vi "Code Complexity String.vi"(11 "CodeComplexity":sgl) -> (3 "Code Complexity String":string)   [LabVIEW 2023, in "VIDoc Printer.lvlib" / "VIDoc Printer.lvclass"]
doc: "Converts the Code Complexity value into a printable String."
uses:
  VIDoc Printer.lvclass
  VIDoc Printer.lvclass/VIDoc Printer.ctl
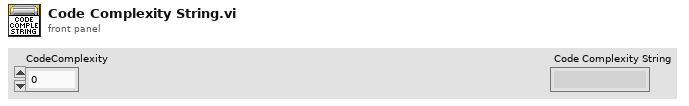
[diagram p1: front panel]
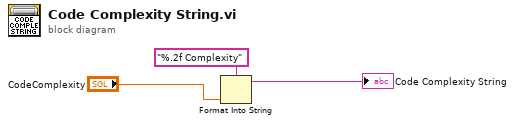
[diagram p0: block diagram]
diagram:
  n1 = Format Into String(format string="%.2f Complexity", "CodeComplexity") -> (resulting string=→"Code Complexity String":string)  [unwired: 2 in, 1 out]
